vi "Trajectory Viewer.vi"(10 "RightDrive":T1={"DeviceStatus"={"status"=FALSE, "code"=0, "source"=""}, "Type"=enum."PWM", "PWM"={"PWM Channel"=enum."Invalid", "DeadBand"={"Name"="", "maxPositivePwm"=0, "minPositivePwm"=0, "centerPwm"=0, "maxNegativePwm"=0, "minNegativePwm"=0, "angularRange"=0}}, "CAN"={"Device Number"=0, "SetOutput VI Ref"=variant(enum8{"Percent VBus", "Current", "Speed", "Position", "Voltage"} enum."Percent VBus"), "GetOutput VI Ref"=variant(refnum<k1> refnum), "Enable VI Ref"=variant(dbl 12.0), "Disable VI Ref"=variant(enum8{"Percent VBus", "Speed", "Position", "Slave", "Unchanged / Invalid", "Voltage Compensation", "Current", "Motion Profile"} enum."Percent VBus"), "Data"=variant}, "Invert"=FALSE, "DIO PWM"={"PWM \"Enable\" Channel"=enum."Invalid", "DIOChannel"=enum."Invalid", "PWM Rate"=0.0}}, 11 "LeftDrive":T1={"DeviceStatus"={"status"=FALSE, "code"=0, "source"=""}, "Type"=enum."PWM", "PWM"={"PWM Channel"=enum."Invalid", "DeadBand"={"Name"="", "maxPositivePwm"=0, "minPositivePwm"=0, "centerPwm"=0, "maxNegativePwm"=0, "minNegativePwm"=0, "angularRange"=0}}, "CAN"={"Device Number"=0, "SetOutput VI Ref"=variant(enum8{"Percent VBus", "Current", "Speed", "Position", "Voltage"} enum."Percent VBus"), "GetOutput VI Ref"=variant(refnum<k1> refnum), "Enable VI Ref"=variant(dbl 12.0), "Disable VI Ref"=variant(enum8{"Percent VBus", "Speed", "Position", "Slave", "Unchanged / Invalid", "Voltage Compensation", "Current", "Motion Profile"} enum."Percent VBus"), "Data"=variant}, "Invert"=FALSE, "DIO PWM"={"PWM \"Enable\" Channel"=enum."Invalid", "DIOChannel"=enum."Invalid", "PWM Rate"=0.0}}) -> ()   [LabVIEW 2018]
uses:
  <vilib>/Rock Robotics/WPI/MotorControl/WPI_MotorControlDeviceRef.ctl
  <vilib>/Rock Robotics/WPI/MotorControl/WPI_MotorControlType.ctl
  <vilib>/Rock Robotics/SystemInterfaces/DIO/FPGA_DIOPWMChannel.ctl
  <vilib>/Rock Robotics/WPI/PWM/WPI_PWMDeadband.ctl
  <vilib>/Rock Robotics/SystemInterfaces/DIO/FPGA_DIOChannel.ctl
  2019_Robot_Code/Subsystems/Drive/driveShifterEnum.ctl
  <vilib>/Rock Robotics/WPI/ThirdParty/Phoenix-LabVIEW/Motor Controller/Get/CTRE_Phoenix_MotorController_GetQuadratureData.vi
panel:
  out "Left Position Error":dbl(graph)
  out "Right Position Error":dbl(graph)
  out "Left Velocity Error":dbl(graph)
  out "Right Velocity Error":dbl(graph)
  out "Velocity (Right)":cluster{dbl, dbl}(graph)
  out "Position (Right)":cluster{"Output":dbl, "Output":dbl}(graph)
  out "Velocity (Left)":cluster{dbl, dbl}(graph)
  out "Position (Left)":cluster{"Output":dbl, "Output":dbl}(graph)
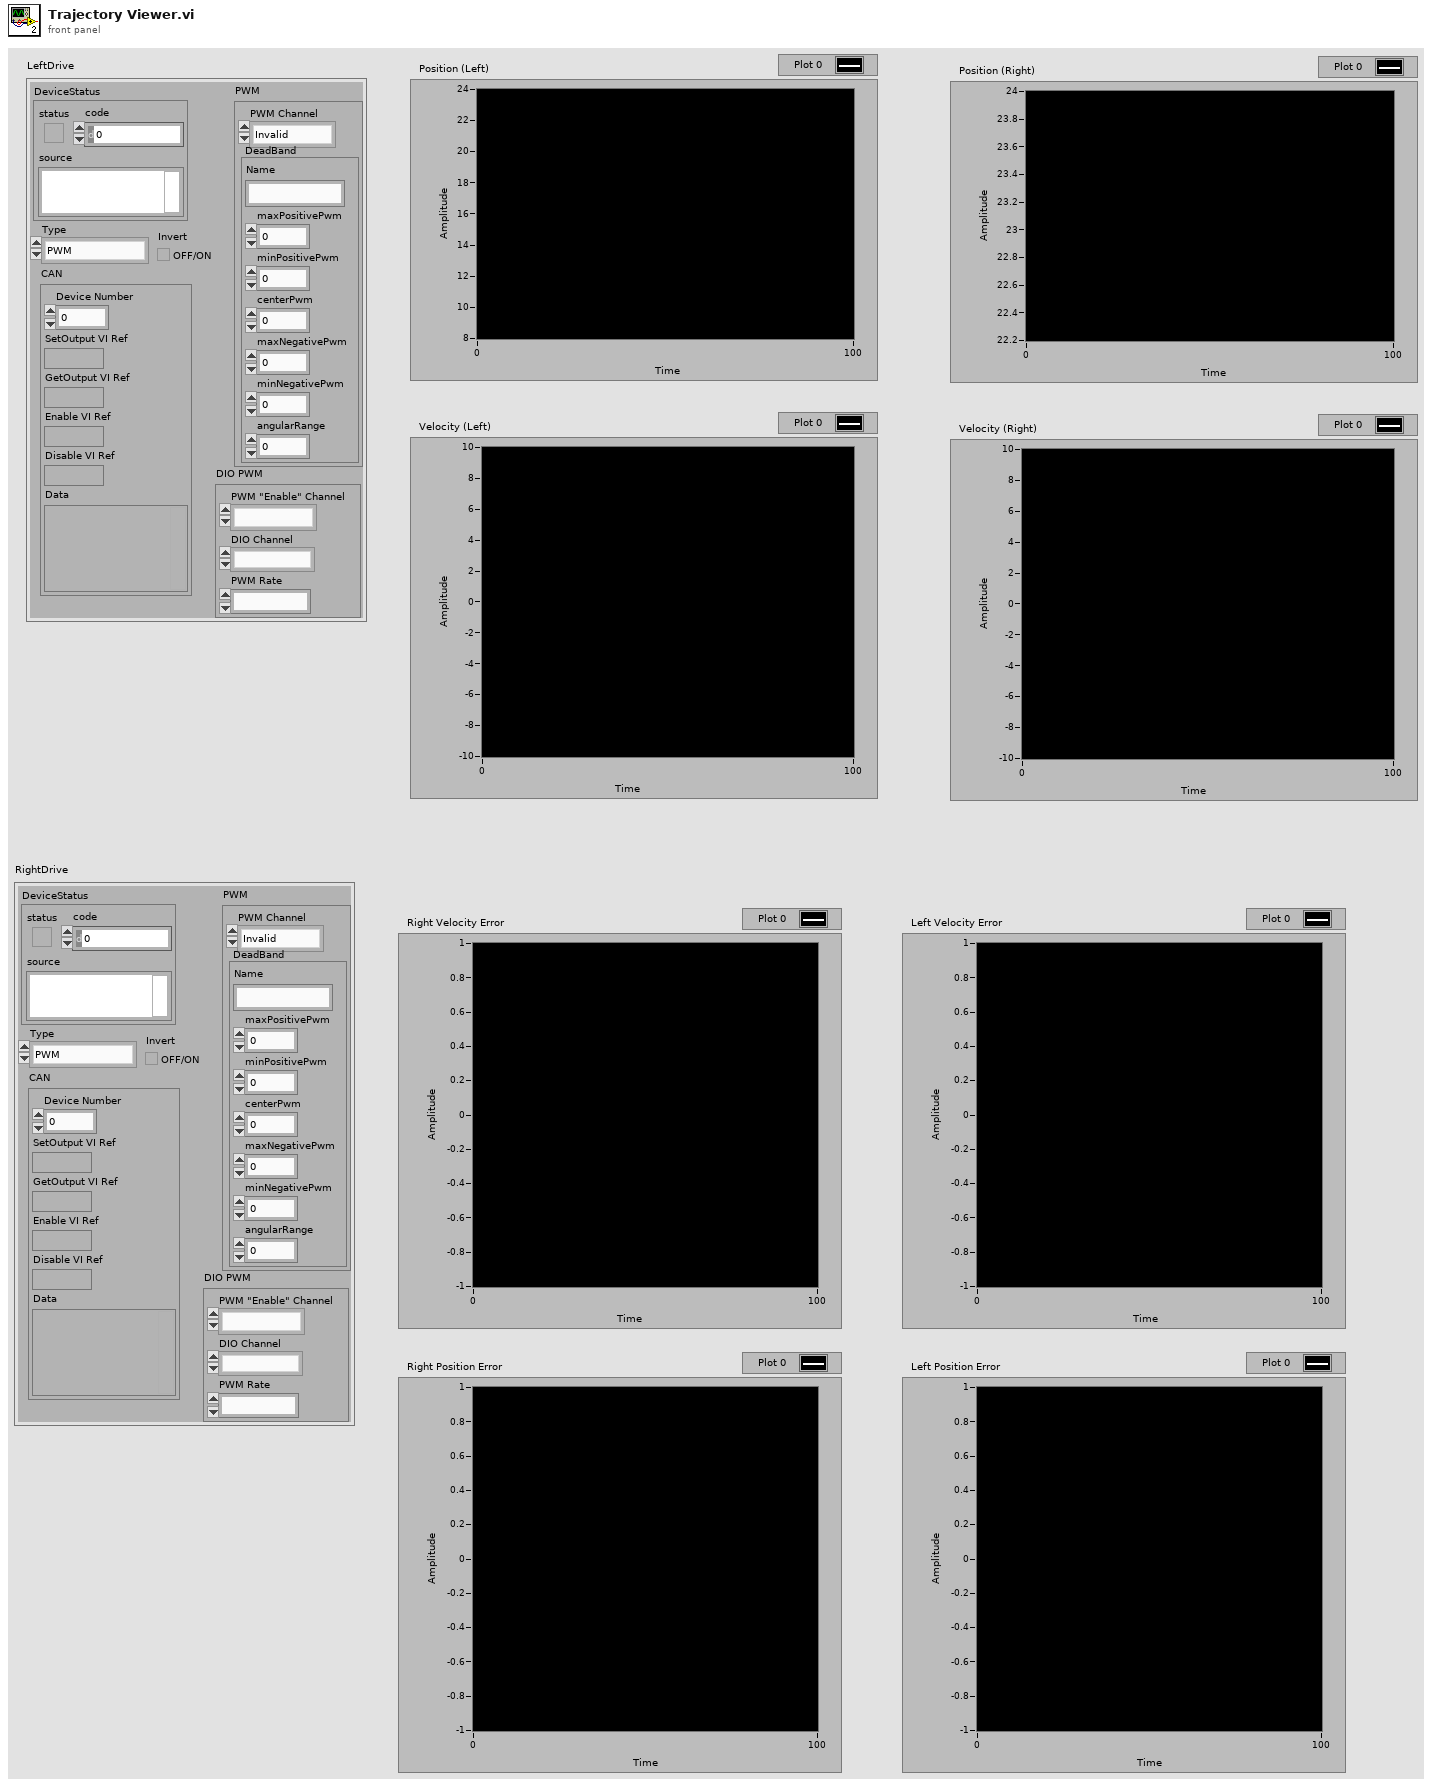
[diagram p1: front panel]
types:
  T1 = typedef "WPI_MotorControlDeviceRef.ctl" = cluster{"DeviceStatus":errorcluster, "Type":T2, "PWM":cluster{"PWM Channel":T3, "DeadBand":T4}, "CAN":cluster{"Device Number":u8, "SetOutput VI Ref":variant, "GetOutput VI Ref":variant, "Enable VI Ref":variant, "Disable VI Ref":variant, "Data":variant}, "Invert":bool, "DIO PWM":cluster{"PWM \"Enable\" Channel":T3, "DIOChannel":T5, "PWM Rate":dbl}}
  T2 = typedef "WPI_MotorControlType.ctl" = enum16{"PWM", "CAN", "DIO PWM"}
  T3 = typedef "FPGA_DIOPWMChannel.ctl" = enum8{"PWM 0", "PWM 1", "PWM 2", "PWM 3", "PWM 4", "PWM 5", "PWM 6", "PWM 7", "PWM 8", "PWM 9", "PWM MXP 0", "PWM MXP 1", "PWM MXP 2", "PWM MXP 3", "PWM MXP 4", "PWM MXP 5", "PWM MXP 6", "PWM MXP 7", "PWM MXP 8", "PWM MXP 9", "Invalid"}
  T4 = typedef "WPI_PWMDeadband.ctl" = cluster{"Name":string, "maxPositivePwm":i32, "minPositivePwm":i32, "centerPwm":i32, "maxNegativePwm":i32, "minNegativePwm":i32, "angularRange":u16}
  T5 = typedef "FPGA_DIOChannel.ctl" = enum8{"DIO 0", "DIO 1", "DIO 2", "DIO 3", "DIO 4", "DIO 5", "DIO 6", "DIO 7", "DIO 8", "DIO 9", "DIO MXP 0", "DIO MXP 1", "DIO MXP 2", "DIO MXP 3", "DIO MXP 4", "DIO MXP 5", "DIO MXP 6", "DIO MXP 7", "DIO MXP 8", "DIO MXP 9", "DIO MXP 10", "DIO MXP 11", "DIO MXP 12", "DIO MXP 13", "DIO MXP 14", "DIO MXP 15", "SPI Port CS1", "SPI Port CS2", "SPI Port CS3", "SPI Port MISO", "SPI Port MOSI", "Invalid"}
  T6 = typedef "driveShifterEnum.ctl" = enum16{"Low", "High"}
  T7 = enum16{"Inches -> Sensor Units", "Sensor Units -> Inches"}
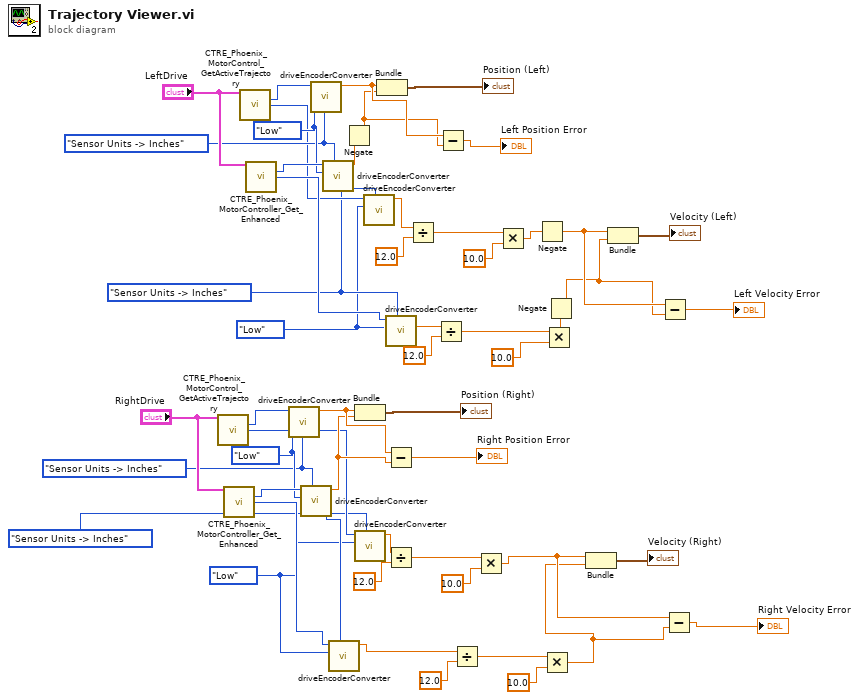
[diagram p0: block diagram]
diagram:
  w3 = driveShifterEnum."Low" ("Gear Setting")
  w5 = T7."Sensor Units -> Inches" ("Conversion Direction")
  w10 = driveShifterEnum."Low" ("Gear Setting")
  w11 = T7."Sensor Units -> Inches" ("Conversion Direction")
  w35 = T7."Sensor Units -> Inches" ("Conversion Direction")
  w36 = driveShifterEnum."Low" ("Gear Setting")
  w50 = T7."Sensor Units -> Inches" ("Conversion Direction")
  w51 = driveShifterEnum."Low" ("Gear Setting")
  n1 = call <vilib>:"CTRE_Phoenix_MotorControl_GetActiveTrajectory.vi"("PhoenixMotorControlDevRef"="RightDrive") -> ("Position (Sensor Units)"=w26:i32, "Velocity (Sensor Units per 100 ms)"=w14:i32)  [unwired: 10 in, 3 out]
  n2 = call-poly <vilib>:"CTRE_Phoenix_MotorController_Get_Enhanced.vi"("PhoenixMotorControlDevRef"="RightDrive") -> ("Quadrature Position"=w37:i32, "Quadrature Velocity"=w12:i32)  [unwired: 11 in, 2 out]
  n3 = call <vilib>:"CTRE_Phoenix_MotorControl_GetActiveTrajectory.vi"("PhoenixMotorControlDevRef"="LeftDrive") -> ("Position (Sensor Units)"=w39:i32, "Velocity (Sensor Units per 100 ms)"=w6:i32)  [unwired: 10 in, 3 out]
  n4 = call-poly <vilib>:"CTRE_Phoenix_MotorController_Get_Enhanced.vi"("PhoenixMotorControlDevRef"="LeftDrive") -> ("Quadrature Position"=w52:i32, "Quadrature Velocity"=w8:i32)  [unwired: 11 in, 2 out]
  n5 = call "driveEncoderConverter.vi"("Conversion Direction"=w35, "Gear Setting"=w36, "Input"=w26) -> ("Output"=w23:dbl)  [unwired: 8 in]
  n6 = call "driveEncoderConverter.vi"("Conversion Direction"=w35, "Gear Setting"=w36, "Input"=w37) -> ("Output"=w22:dbl)  [unwired: 8 in]
  n7 = call "driveEncoderConverter.vi"("Conversion Direction"=w50, "Gear Setting"=w51, "Input"=w39) -> ("Output"=w21:dbl)  [unwired: 8 in]
  n8 = call "driveEncoderConverter.vi"("Conversion Direction"=w50, "Gear Setting"=w51, "Input"=w52) -> ("Output"=w41:dbl)  [unwired: 8 in]
  n9 = call "driveEncoderConverter.vi"("Conversion Direction"=w11, "Gear Setting"=w10, "Input"=w12) -> ("Output"=w9:dbl)  [unwired: 8 in]
  n10 = Negate(x=w41) -> (-x=w20:dbl)
  n11 = Bundle("Output"=w23, "Output"=w22) -> (→"Position (Right)":cluster{"Output":dbl, "Output":dbl})  [unwired: 1 in]
  n12 = call "driveEncoderConverter.vi"("Conversion Direction"=w11, "Gear Setting"=w10, "Input"=w14) -> ("Output"=w13:dbl)  [unwired: 8 in]
  n13 = call "driveEncoderConverter.vi"("Conversion Direction"=w5, "Gear Setting"=w3, "Input"=w6) -> ("Output"=w4:dbl)  [unwired: 8 in]
  n14 = Bundle("Output"=w21, w20) -> (→"Position (Left)":cluster{"Output":dbl, dbl})  [unwired: 1 in]
  n15 = call "driveEncoderConverter.vi"("Conversion Direction"=w5, "Gear Setting"=w3, "Input"=w8) -> ("Output"=w7:dbl)  [unwired: 8 in]
  n16 = Subtract(x=w23, y=w22) -> (x-y=→"Right Position Error":dbl)
  n17 = Divide(x=w13, y=12.0) -> (x/y=w31:dbl)
  n18 = Divide(x=w4, y=12.0) -> (x/y=w46:dbl)
  n19 = Divide(x=w7, y=12.0) -> (x/y=w43:dbl)
  n20 = Subtract(x=w21, y=w20) -> (x-y=→"Left Position Error":dbl)
  n21 = Divide(x=w9, y=12.0) -> (x/y=w28:dbl)
  n22 = Multiply(x=w31, y=10.0) -> (x*y=w25:dbl)
  n23 = Multiply(x=w46, y=10.0) -> (x*y=w40:dbl)
  n24 = Negate(x=w40) -> (-x=w19:dbl)
  n25 = Multiply(x=w28, y=10.0) -> (x*y=w24:dbl)
  n26 = Multiply(x=w43, y=10.0) -> (x*y=w2:dbl)
  n27 = Negate(x=w2) -> (-x=w1:dbl)
  n28 = Bundle(w25, w24) -> (→"Velocity (Right)":cluster{dbl, dbl})  [unwired: 1 in]
  n29 = Bundle(w19, w1) -> (→"Velocity (Left)":cluster{dbl, dbl})  [unwired: 1 in]
  n30 = Subtract(x=w19, y=w1) -> (x-y=→"Left Velocity Error":dbl)
  n31 = Subtract(x=w25, y=w24) -> (x-y=→"Right Velocity Error":dbl)
